vi "CRYASIOGetNumDrivers.vi"(11 "error in (no error)":errorcluster) -> (0 "Drive Num":i32, 3 "error out":errorcluster)   [LabVIEW 2013]
uses:
  CRY_ASIO.dll
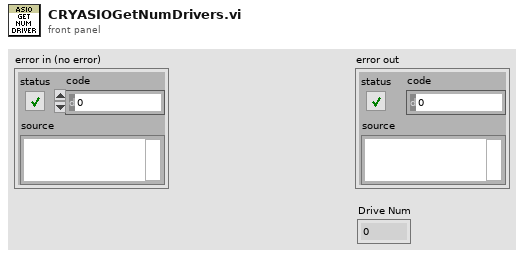
[diagram p1: front panel]
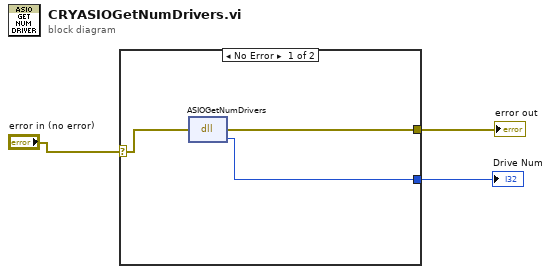
[diagram p0: block diagram]
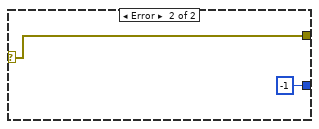
[diagram p2: hidden frame]
diagram:
  n1 = case shown="No Error" "error in (no error)" {
    selector: "error in (no error)" -> [w4 w8]
    tunnel: [w6 -1 ("return type")] -> w2
    tunnel: [w5 w8] -> w1
    frame No Error {
      n2 = dll-call lib="D:/LabView_Project/CRY6181/CRY_ASIO.dll" fn="ASIOGetNumDrivers"(error in=w4) -> (error out=w5:errorcluster, "return type"=w6:i32)  [unwired: 2 in, 1 out]
    }
    frame Error {
    }
  }
  "Drive Num" <- w2
  "error out" <- w1
